vi "Test Reponse.vi"() -> ()   [LabVIEW 2016]
uses:
  WebSocket Server/Http Response Codes.ctl
  WebSocket Server/WebSocket Server.lvclass
panel:
  in  "Http Response Codes":T1=403 items=["Forbidden"=403, "Not Found"=404, "Upgrade Required"=426]
  out "Status Code":T1 items=["Forbidden"=403, "Not Found"=0, "Upgrade Required"=426]
  out "Reason-Phrase":string
  out "Http Version":string
  out "Headers Array":string[][](array[string])
  out "HTTP Request":string
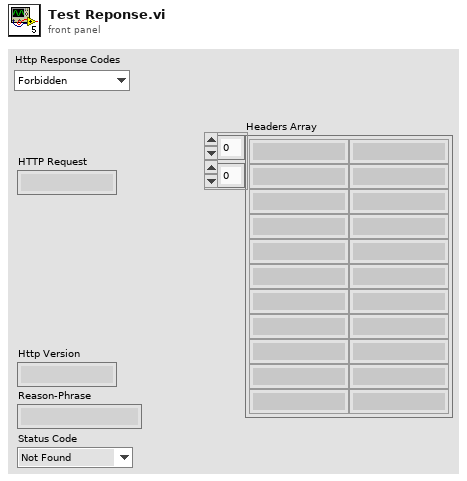
[diagram p1: front panel]
types:
  T1 = typedef "WebSocket Actors.lvlib/WebSocket Server.lvclass/Http Response Codes.ctl" = u16
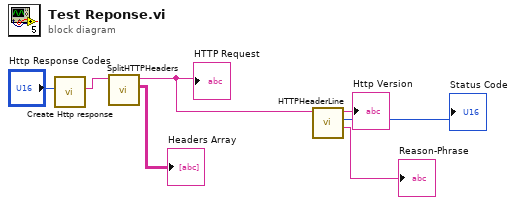
[diagram p0: block diagram]
diagram:
  n1 = call "Create Http response.vi"("Http Response Codes"="Http Response Codes") -> ("Http Response"=w2:string)  [unwired: 10 in]
  n2 = call "SplitHTTPHeaders.vi"("HTTP Header String"=w2) -> ("Headers Array"=→"Headers Array":string[][], "HTTP Request"=w6:string)  [unwired: 8 in, 1 out]
  "HTTP Request" <- w6
  n3 = call "HTTPHeaderLine.vi"("HTTP Request Line"=w6) -> ("Reason-Phrase"=→"Reason-Phrase":string, "Status Code"=→"Status Code":T1, "Http Version"=→"Http Version":string)  [unwired: 7 in, 1 out]
